vi "PH_SHS_Analysis.ProcEvents.vi"(0 "i ref in":refnum<vi>, 5 "error in":errorcluster) -> (14 "i ref out":refnum<vi>, 19 "error out":errorcluster)   [LabVIEW 2014, in "PH_SHS_Analysis.lvlib"]
doc: "This method is used to define the events the object will listen to. Add your own events here."
uses:
  PH_SHS_Analysis.lvlib
  CSCore/BaseProcess/BaseProcess.event definition.ctl
  CSCore/CAEObj/CAEObj.event definition.ctl
  CSCore/BaseProcess/BaseProcess.descriptor string definition.ctl
  CSCore/BaseProcess/BaseProcess.lvlib
  CSCore/CAEObj/CAEObj.lvlib
  PH_Common/PH_Common.lvlib
  PH_Img_BaseClass/PH_Img_BaseClass.lvlib
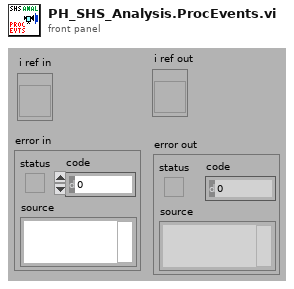
[diagram p1: front panel]
types:
  T1 = typedef "BaseProcess.lvlib/BaseProcess.event definition.ctl" = cluster{"CAEEvtDef":T2, "Data Descriptor":T3}
  T2 = typedef "CAEObj.lvlib/CAEObj.event definition.ctl" = cluster{"URL":string, "enable":bool, "ignoreResID":bool}
  T3 = typedef "BaseProcess.lvlib/BaseProcess.descriptor string definition.ctl" = string
  T4 = typedef "PH_Img_BaseClass.lvlib/PH_Img_BaseClass.i attribute.ctl" = cluster{"GUI Refs":T5, "Timeout Image [ms]":i32, "Default Periodic Period [ms]":i32, "Camera":cluster{"Instancename":string, "Notifier":refnum<notifier>}, "Palette":T6, "Cam Settings":cluster{"Cam ID":string, "Gain":dbl, "Brightness":dbl, "Shutter":dbl, "Cam Info Failure":bool, "Mode":i32}}
  T5 = typedef "PH_Img_BaseClass.lvlib/PH_Img_BaseClass.GUI Refs.ctl" = cluster{"Timeout":refnum<vi>, "Image":refnum<vi>, "Palette":refnum<vi>, "Timeout Set":refnum<vi>}
  T6 = typedef "PH_Img_BaseClass.lvlib/PH_Img_BaseClass.Palette.ctl" = i32
  T7 = typedef "PH_Common.lvlib/PH_DIM.Event Declarer.ctl" = cluster{"Service Name":string, "Selector":string}
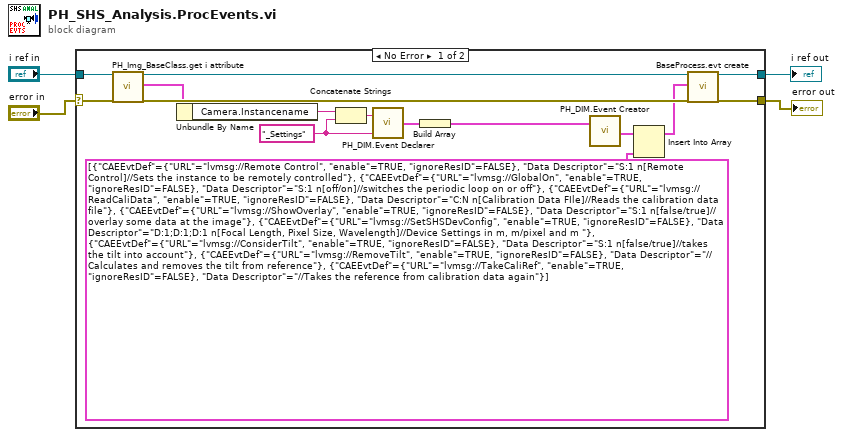
[diagram p0: block diagram]
diagram:
  n1 = case shown="No Error" "error in" {
    selector: "error in" -> [w17 w20]
    tunnel: "i ref in" -> [w15 w21]
    tunnel: [w19 w21] -> w3
    tunnel: [w18 w20] -> w2
    frame No Error {
      w9 = "_Settings" ("Service Name")
      n2 = call "PH_Img_BaseClass.get i attribute.vi"("i ref in"=w15, "error in (no error)"=w17) -> ("i ref out"=w14:refnum<vi>, "i attribute"=w7:T4, "error out"=w16:errorcluster)  [unwired: 15 in]
      n3 = Unbundle By Name(w7) -> ("Camera.Instancename"=w5:string)
      n4 = Concatenate Strings(w5, w9) -> (w8:string)
      n5 = call "PH_DIM.Event Declarer.vi"("Selector"=w9, "Service Name"=w8) -> ("declared DIM Event"=w10:T7)
      n6 = Build Array(w10) -> (w6:T7[])
      n7 = call "PH_DIM.Event Creator.vi"("Trendmessage Services"=w6) -> ("DIM Service Events"=w11:T1[])  [unwired: 18 in]
      n8 = Insert Into Array(array=w11, new element=T1[] [{"CAEEvtDef"={"URL"="lvmsg://Remote Control", "enable"=TRUE, "ignoreResID"=FALSE}, "Data Descriptor"="S:1 n[Remote Control]//Sets the instance to be remotely controlled"}, {"CAEEvtDef"={"URL"="lvmsg://GlobalOn", "enable"=TRUE, "ignoreResID"=FALSE}, "Data Descriptor"="S:1 n[off/on]//switches the periodic loop on or off"}, {"CAEEvtDef"={"URL"="lvmsg://ReadCaliData", "enable"=TRUE, "ignoreResID"=FALSE}, "Data Descriptor"="C:N n[Calibration Data FIle]//Reads the calibration data file"}, {"CAEEvtDef"={"URL"="lvmsg://ShowOverlay", "enable"=TRUE, "ignoreResID"=FALSE}, "Data Descriptor"="S:1 n[false/true]//overlay some data at the image"}, {"CAEEvtDef"={"URL"="lvmsg://SetSHSDevConfig", "enable"=TRUE, "ignoreResID"=FALSE}, "Data Descriptor"="D:1;D:1;D:1 n[Focal Length, Pixel Size, Wavelength]//Device Settings in m, m/pixel and m "}, {"CAEEvtDef"={"URL"="lvmsg://ConsiderTilt", "enable"=TRUE, "ignoreResID"=FALSE}, "Data Descriptor"="S:1 n[false/true]//takes the tilt into account"}, {"CAEEvtDef"={"URL"="lvmsg://RemoveTilt", "enable"=TRUE, "ignoreResID"=FALSE}, "Data Descriptor"="//Calculates and removes the tilt from reference"}, {"CAEEvtDef"={"URL"="lvmsg://TakeCaliRef", "enable"=TRUE, "ignoreResID"=FALSE}, "Data Descriptor"="//Takes the reference from calibration data again"}] ("new events")) -> (w13:T1[])  [unwired: 1 in]
      n9 = call "BaseProcess.evt create.vi"("i ref in"=w14, "newEvents"=w13, "error in (no error)"=w16) -> ("i ref out"=w19:refnum<vi>, "error out"=w18:errorcluster)  [unwired: 13 in, 2 out]
    }
    frame Error {
    }
  }
  "i ref out" <- w3
  "error out" <- w2
